vi "2015myGlobal 1.vi"() -> ()   [LabVIEW 2012]
panel:
  in  "停留時間(秒)":dbl=4.0
  in  "Fource_LoadCell (V)":dbl=4.0
  in  "步進馬達位置":i32=4
  in  "重複次數":i32=4
  in  "速度參數":i32
  in  "前進STEP":i32
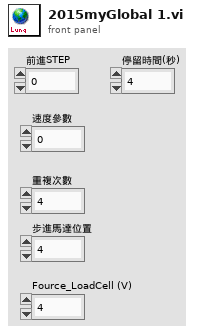
[diagram p1: front panel]
diagram:
